vi "from.Bytes.vi"(8 "error in (no error)":errorcluster, 10 "Bytes.In":u8[](array[numeric]) format="%.0x", 11 "SequencedUnitHeader in":refnum<class "SequencedUnitHeader.lvclass">) -> (0 "error out":errorcluster, 2 "Remaining Bytes":u8[](array[numeric]), 3 "SequencedUnitHeader out":refnum<class "SequencedUnitHeader.lvclass">)   [LabVIEW 2020, in "SequencedUnitHeader.lvclass"]
uses:
  SequencedUnitHeader.lvclass
panel:
  out "subset deleted":u8[](array[numeric]) format="%.0x"
  out "First Seq":u32
  out "Next Seq":u32 format="%.0x"
  out "Hdr Length":u16 format="%.0x"
  out "Hdr Count":u8 format="%.0x"
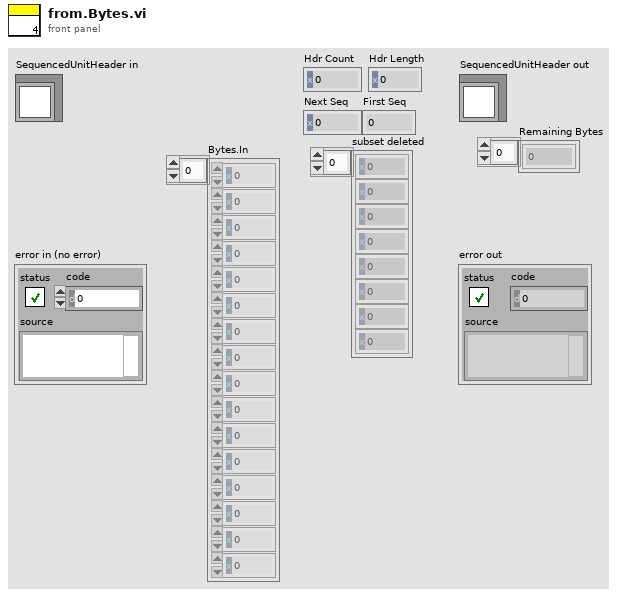
[diagram p1: front panel]
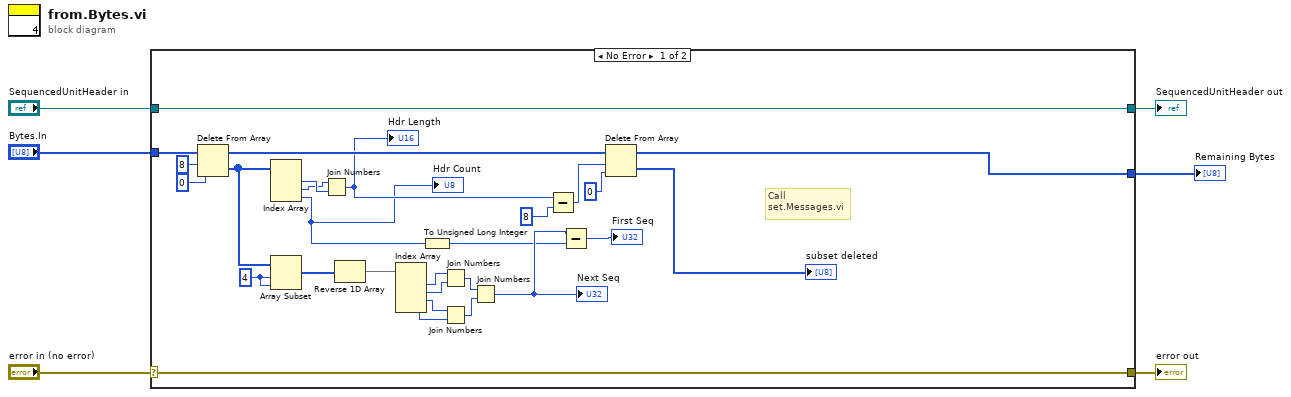
[diagram p0: block diagram]
diagram:
  n1 = case shown="No Error" "error in (no error)" {
    selector: "error in (no error)" -> [w33 w37]
    tunnel: [w33 w37] -> w5
    tunnel: [w34 w36] -> w3
    tunnel: "SequencedUnitHeader in" -> [w34 w36]
    tunnel: "Bytes.In" -> [w32 w35]
    tunnel: [w9 w35] -> w1
    frame No Error {
      w26 = 4 ("index")
      # "Call\nset.Messages.vi"
      n2 = Delete From Array(array=w32, length=8, index=0) -> (deleted portion=w27:u8[], array with subset deleted=w15:u8[])
      n3 = Index Array(array=w27) -> (element #1=w29:u8, element #2=w28:u8, element #3=w8:u8)  [unwired: 3 in]
      "Hdr Count" <- w8
      n4 = Array Subset(array=w27, index=w26, length=w26) -> (w25:u8[])
      n5 = Join Numbers(hi=w28, lo=w29) -> ((hi.lo)=w11:u16)
      "Hdr Length" <- w11
      n6 = Reverse 1D Array(array=w25) -> (reversed array=w24:u8[])
      n7 = Index Array(array=w24) -> (element #1=w23:u8, element #2=w22:u8, element #3=w21:u8, element #4=w20:u8)  [unwired: 4 in]
      n8 = To Unsigned Long Integer(number=w8) -> (unsigned 32bit integer=w7:u32)
      n9 = Join Numbers(hi=w23, lo=w22) -> ((hi.lo)=w18:u16)
      n10 = Join Numbers(hi=w21, lo=w20) -> ((hi.lo)=w19:u16)
      n11 = Join Numbers(hi=w18, lo=w19) -> ((hi.lo)=w17:u32)
      "Next Seq" <- w17
      n12 = Subtract(x=w11, y=u8 8) -> (x-y=w13:u16)
      n13 = Subtract(x=w17, y=w7) -> (x-y=→"First Seq":u32)
      n14 = Delete From Array(array=w15, length=w13, index=0) -> (deleted portion=→"subset deleted":u8[], array with subset deleted=w9:u8[])
    }
    frame Error {
    }
  }
  "error out" <- w5
  "SequencedUnitHeader out" <- w3
  "Remaining Bytes" <- w1
